vi "Gamma PDF.vi"(9 "c":dbl=1.0, 10 "b":dbl=1.0, 11 "x":dbl=0.5) -> (0 "error":i32, 3 "pdf(x)":dbl=0.6065306597126334)   [LabVIEW 2020, in "NI_Gmath.lvlib"]
doc: "Computes the continuous probability density function (PDF) of various distributions. You must manually select the polymorphic instance to use."
uses:
  NI_Gmath.lvlib
  st_error_code.ctl
  Gamma Function.vi
panel:
  # "Gamma PDF"
  # "scale"
  # "shape"
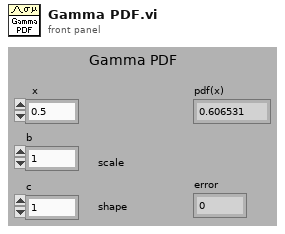
[diagram p1: front panel]
types:
  T1 = typedef "NI_Gmath.lvlib/st_error_code.ctl" = i32
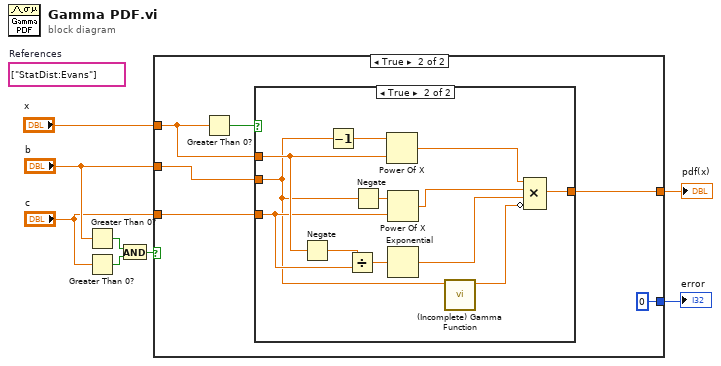
[diagram p0: block diagram]
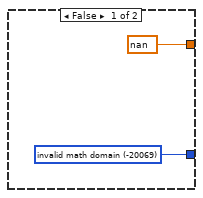
[diagram p2: hidden frame]
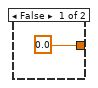
[diagram p3: hidden frame]
diagram:
  (unwired) string[] ["StatDist:Evans"]  # References
  n1 = Greater Than 0?(x="b") -> (x > 0?=w3:bool)
  n2 = Greater Than 0?(x="c") -> (x > 0?=w4:bool)
  n3 = And(x=w3, y=w4) -> (x .and. y?=w5:bool)
  n4 = case shown="True" w5 {
    tunnel: "c" -> [_ w13]
    tunnel: [w9 0 ("invalid math domain")] -> w8
    tunnel: [nan w15] -> w7
    tunnel: "x" -> [_ w12]
    tunnel: "b" -> [_ w14]
    frame False {
      w9 = T1 -20069 items=["invalid math domain"=-20069, "Fourier interpolation size m >= n"=-20070, "empty array"=-20003] ("stat interp error code")
    }
    frame True {
      n5 = Greater Than 0?(x=w12) -> (x > 0?=w11:bool)
      n6 = case shown="True" w11 {
        tunnel: [0.0 w18] -> w15
        tunnel: w12 -> [_ w26]
        tunnel: w14 -> [_ w23]
        tunnel: w13 -> [_ w25]
        frame False {
        }
        frame True {
          n7 = Negate(x=w26) -> (-x=w27:dbl)
          n8 = Decrement(x=w23) -> (x-1=w29:dbl)
          n9 = Divide(x=w27, y=w25) -> (x/y=w24:dbl)
          n10 = Negate(x=w23) -> (-x=w28:dbl)
          n11 = Power Of X(1:w26, 2:w29) -> (0:w22:dbl)
          n12 = Power Of X(1:w25, 2:w28) -> (0:w21:dbl)
          n13 = Exponential(1:w24) -> (0:w20:dbl)
          n14 = call-poly "(Incomplete) Gamma Function.vi"("x"=w23) -> ("g(x)"=w19:dbl)  [unwired: 10 in]
          n15 = Compound Arithmetic op=MULTIPLY(w22, w21, w20, invert w19) -> (w18:dbl)
        }
      }
    }
  }
  "pdf(x)" <- w7
  "error" <- w8
